vi "Config - CheckIfMeasurementActive.vi"(8 "Fehler (Eingang, kein Fehler)":errorcluster) -> (0 "Fehler (Ausgang)":errorcluster)   [LabVIEW 2009]
uses:
  eGateUtility.dll
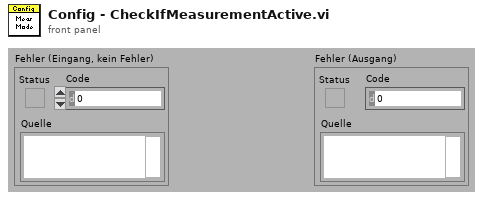
[diagram p1: front panel]
types:
  T1 = enum16{"open", "replace", "create", "open or create", "replace or create", "replace or create with confirmation"}
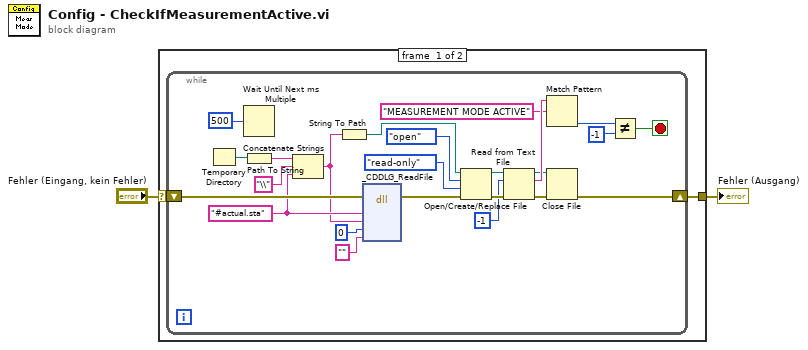
[diagram p0: block diagram]
diagram:
  n1 = case shown="Kein Fehler" "Fehler (Eingang, kein Fehler)" {
    selector: "Fehler (Eingang, kein Fehler)" -> [w3 w29]
    tunnel: [w4 w29] -> w2
    frame #0 {
      n2 = while {
        shift-right: [w7] -> w4
        shift-left: w3 -> [w28]
        stop <- w10 stop-if-true
        w27 = "#actual.sta" ("SourceFileName")
        n3 = Temporary Directory() -> (w6:path)
        n4 = Wait Until Next ms Multiple(millisecond multiple=u32 500 ("Vielfache von ms")) -> ()  [unwired: 1 out]
        n5 = Path To String(path=w6) -> (string=w5:string)
        n6 = Concatenate Strings(w5, "\\" ("String"), w27) -> (w22:string)
        n7 = String To Path(string=w22) -> (path=w21:path)
        n8 = dll-call lib="eGateUtility.dll" fn="_CDDLG_ReadFile"(error in=w28, "SourceFileName"=w27, "DestinationFullFileName"=w22, "AppendToExisting"=0, "ErrorString"="") -> (error out=w23:errorcluster)  [unwired: 4 in, 4 out]
        n9 = Open/Create/Replace File(file path (use dialog)=w21, error in=w23, operation (0:open)=T1."open" ("Operation (0:Öffnen)"), access (0:read/write)=enum16{"read/write", "read-only", "write-only"}."read-only" ("Zugriff (0:Lesen/Schreiben)")) -> (refnum out=w18:refnum<file>, error out=w17:errorcluster)  [unwired: 3 out]
        n10 = Read from Text File(file (use dialog)=w18, count=-1 ("Anzahl"), error in=w17) -> (refnum out=w8:refnum<file>, text=w14:string, error out=w9:errorcluster)  [unwired: 2 out]
        n11 = Match Pattern(string=w14, regular expression="MEASUREMENT MODE ACTIVE" ("Regulärer Ausdruck")) -> (offset past match=w12:i32)  [unwired: 4 out]
        n12 = Close File(refnum=w8, error in=w9) -> (error out=w7:errorcluster)  [unwired: 1 out]
        n13 = Not Equal?(x=w12, y=-1) -> (x != y?=w10:bool)
      }
    }
    frame #1 {
    }
  }
  "Fehler (Ausgang)" <- w2
